vi "receiver.vi"(5 "Sync Words":i32[](array[numeric]), 7 "preamble length":i32, 8 "error in (no error)":errorcluster, 9 "Key Bit Sequence":u32[](array[numeric]), 10 "input complex waveform":cluster{"t0":dbl, "dt":dbl, "Y":cdb[]}, 11 "Modulation Parameters In":T1={"RX Parameters"={"RX Oversample Factor"=4, "RX Sample Rate"=4000000.0, "Synchronization Options"={"Synchronization Method"=enum."Fixed Offset", "Symbol Timing Recovery Method "=enum."MT Allign To Ideal Symbols", "Fixed Offset"=0.0, "Frame Detection Method"=enum."", "Correct Frequency Offset"=FALSE}, "Channel Estimation/Equalization Parameters"={"Equalization Method"=enum."", "Channel Estimate Length"=0.0, "Equalizer Length"=0.0, "Equalizer Delay"=0.0}}, "TX/RX Shared Parameters"={"Modulation Type"=enum."OOK", "Packet Length"=128, "# of Iterations"=0.0, "Pulse Shaping Parameters"={"Pulse Shaping Filter"=enum."none", "Filter Length (symbols)"=32, "Filter Parameter"=0.8, "modulation type"=enum."FSK"}, "Header/Tail Control Information"={"Training Sequence Type"=enum."", "Zero Pad Length"=0.0}}}) -> (0 "error out":errorcluster, 2 "recovered bits":i32[](array[numeric]), 3 "BER":dbl, 4 "Recovered Symbols":cdb[](array[numeric]))   [LabVIEW 2012]
panel:
  out "theta":dbl[](array[numeric])
  out "r":dbl[](array[numeric])
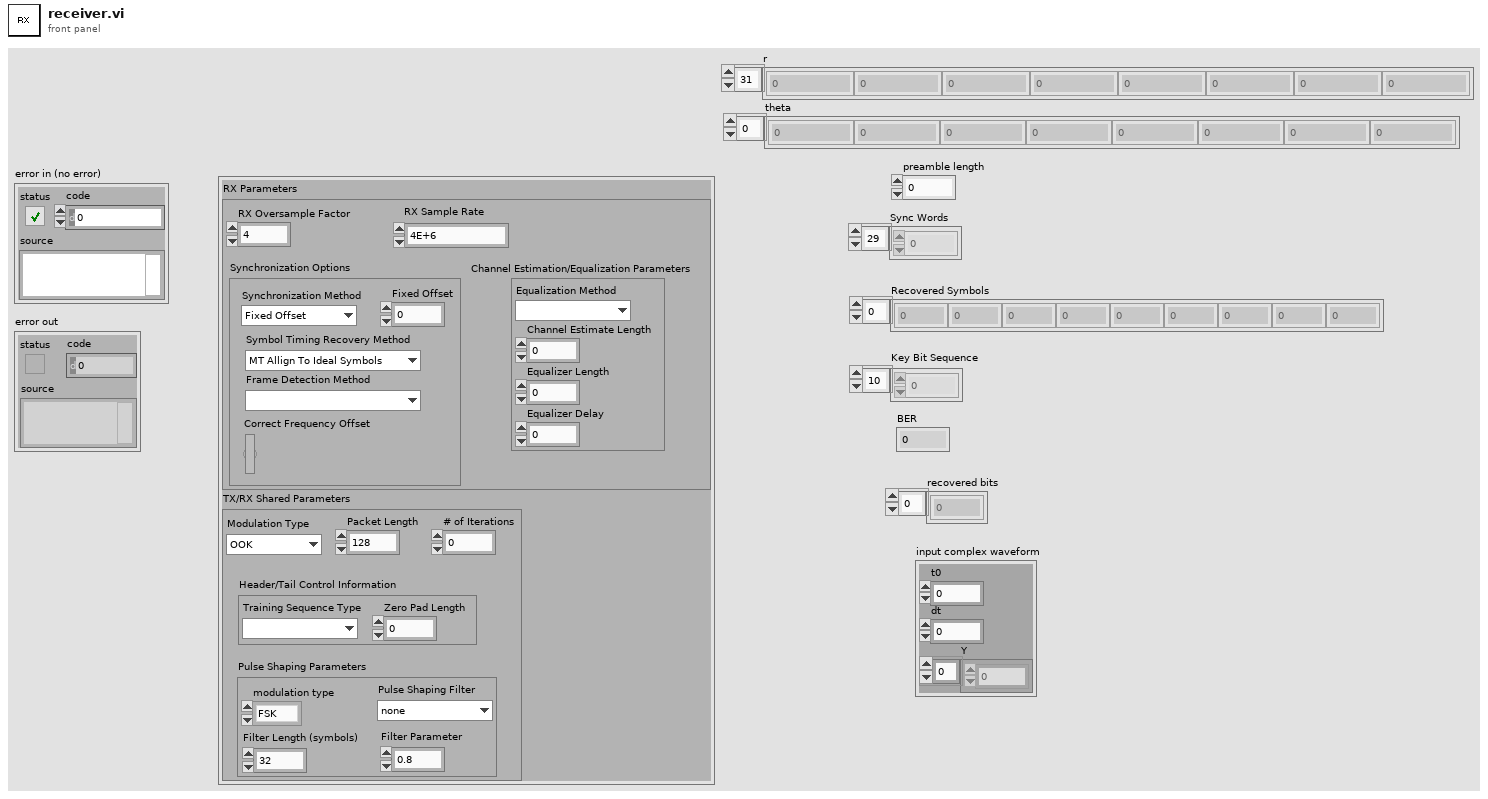
[diagram p1: front panel]
types:
  T1 = cluster{"RX Parameters":cluster{"RX Oversample Factor":i32, "RX Sample Rate":dbl, "Synchronization Options":cluster{"Synchronization Method":enum16{"Fixed Offset", "Timing Estimation", "Joint Timing and Channel Estimation"}, "Symbol Timing Recovery Method ":enum16{"MT Allign To Ideal Symbols", "Maximum Energy", "Early-Late Gate", "Gardner", "Fixed Offset"}, "Fixed Offset":dbl, "Frame Detection Method":enum16{""}, "Correct Frequency Offset":bool}, "Channel Estimation/Equalization Parameters":cluster{"Equalization Method":enum16{""}, "Channel Estimate Length":dbl, "Equalizer Length":dbl, "Equalizer Delay":dbl}}, "TX/RX Shared Parameters":cluster{"Modulation Type":enum16{"OOK", "FSK"}, "Packet Length":i32, "# of Iterations":dbl, "Pulse Shaping Parameters":cluster{"Pulse Shaping Filter":enum16{"none", "Raised Cosine", "Root Raised Cos", "Gaussian"}, "Filter Length (symbols)":i32, "Filter Parameter":dbl, "modulation type":enum16{"FSK", "PSK", "QAM", "MSK", "PAM", "ASK", "CPM"}}, "Header/Tail Control Information":cluster{"Training Sequence Type":enum16{""}, "Zero Pad Length":dbl}}}
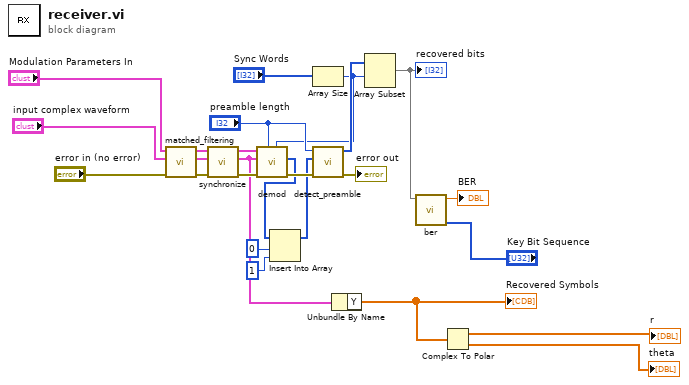
[diagram p0: block diagram]
diagram:
  n1 = call "matched_filtering.vi"("error in (no error)"="error in (no error)", "input complex waveform"="input complex waveform", "Modulation Parameters In"="Modulation Parameters In") -> ("error out"=w14:errorcluster, "output complex waveform"=w15:cluster{"t0":dbl, "dt":dbl, "Y":cdb[]}, "Modulation Parameters Out"=w16:T1)  [unwired: 6 in]
  n2 = call "synchronize.vi"("error in (no error)"=w14, "input complex waveform"=w15, "Modulation Parameters In"=w16) -> ("error out"=w12:errorcluster, "output complex waveform"=w10:cluster{"t0":dbl, "dt":dbl, "Y":cdb[]}, "Modulation Parameters Out"=w13:T1)  [unwired: 6 in]
  n3 = Array Size(array="Sync Words") -> (size(s)=w2:i32)
  n4 = call "demod.vi"("Sync Word Length"=w2, "Preamble Length"="preamble length", "error in (no error)"=w12, "input complex waveform"=w10, "Modulation Parameters In"=w13) -> ("error out"=w11:errorcluster, "Received Bit Sequence"=w6:i32[])  [unwired: 4 in, 1 out]
  n5 = Insert Into Array(array=w6, index=0, new element=1 ("new element/subarray")) -> (w1:i32[])
  n6 = call "detect_preamble.vi"("error in (no error)"=w11, "Recovered Bit Sequence"=w1, "preamble length"="preamble length") -> ("error out"=→"error out":errorcluster, "Bit Sequence"=w24:i32[])  [unwired: 7 in]
  n7 = Unbundle By Name(w10) -> ("Y"=w9:cdb[])
  "Recovered Symbols" <- w9
  n8 = Array Subset(array=w24, index=w2) -> (w23:i32[])  [unwired: 1 in]
  "recovered bits" <- w23
  n9 = call "ber.vi"("Key Bit Sequence"="Key Bit Sequence", "Recovered Bit Sequence"=w23) -> ("BER"=→"BER":dbl)  [unwired: 9 in]
  n10 = Complex To Polar(r * e^(i*theta)=w9) -> (r=→"r":dbl[], theta=→"theta":dbl[])
